vi "Create User Events.vi"(8 "error in (no error)":errorcluster, 11 "Helper Loop in":refnum<class "Helper Loop.lvclass">) -> (0 "error out":errorcluster, 3 "Helper Loop out":refnum<class "Helper Loop.lvclass">)   [LabVIEW 2024, in "Helper Loop.lvlib" / "Helper Loop.lvclass"]
uses:
  Helper Loop.lvclass
  Helper Loop.lvclass/Helper Loop.ctl
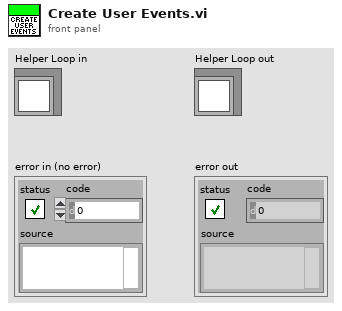
[diagram p1: front panel]
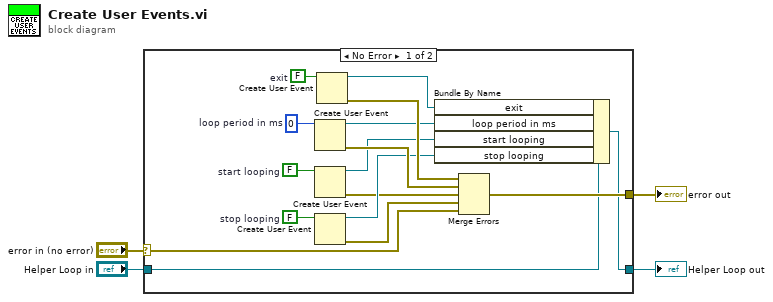
[diagram p0: block diagram]
diagram:
  n1 = case shown="No Error" "error in (no error)" {
    selector: "error in (no error)" -> [w5 w22]
    tunnel: [w16 w22] -> w3
    tunnel: [w12 w21] -> w1
    tunnel: "Helper Loop in" -> [w15 w21]
    frame No Error {
      w10 = FALSE  # stop looping
      w11 = FALSE  # start looping
      w19 = u32 0  # loop period in ms
      w20 = FALSE  # exit
      n2 = Create User Event(user event datatype=w19) -> (user event=w13:refnum<user-event>, error out=w17:errorcluster)  [unwired: 1 in]
      n3 = Create User Event(user event datatype=w11) -> (user event=w9:refnum<user-event>, error out=w7:errorcluster)  [unwired: 1 in]
      n4 = Create User Event(user event datatype=w10) -> (user event=w8:refnum<user-event>, error out=w6:errorcluster)  [unwired: 1 in]
      n5 = Create User Event(user event datatype=w20) -> (user event=w14:refnum<user-event>, error out=w18:errorcluster)  [unwired: 1 in]
      n6 = Bundle By Name(cluster=w15, "exit"=w14, "loop period in ms"=w13, "start looping"=w9, "stop looping"=w8) -> (w12:refnum<class "Helper Loop.lvclass">)
      n7 = Merge Errors(w18, w17, w7, w6, w5) -> (w16:errorcluster)
    }
    frame Error {
    }
  }
  "error out" <- w3
  "Helper Loop out" <- w1
